vi "Pusher_Client_SetHandler.vi"(6 "_data":T1, 8 "ErrIn":errorcluster, 9 "Debug(F)":bool, 11 "Client in":refnum<class "Client.lvclass">) -> (0 "ErrOut":errorcluster, 2 "Path":path, 3 "Client out":refnum<class "Client.lvclass">)   [LabVIEW 2009, in "Client.lvclass"]
uses:
  Client.lvclass
  Pusher_Client_MonitorData.ctl
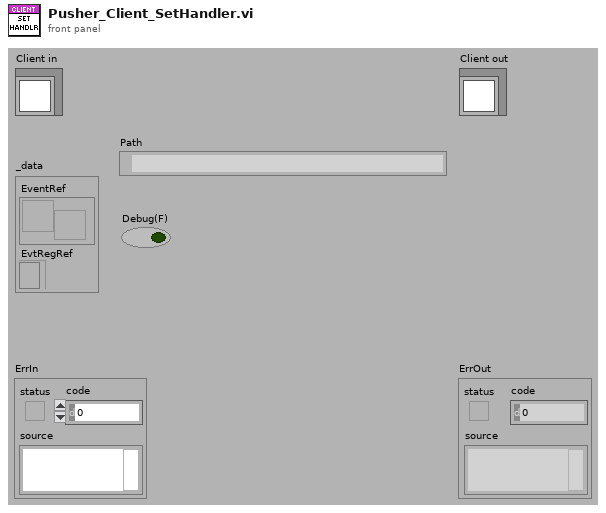
[diagram p1: front panel]
types:
  T1 = typedef "Client.lvclass/Pusher_Client_MonitorData.ctl" = cluster{"EventRef":refnum<user-event>, "EvtRegRef":refnum<event-registration>}
  T2 = enum32{"Invalid", "Standard", "Closed", "Hidden", "Minimized", "Maximized"}
  T3 = enum32{"Bad", "Idle", "Run top level", "Running"}[]
  T4 = enum32{"Bad", "Idle", "Run top level", "Running"}
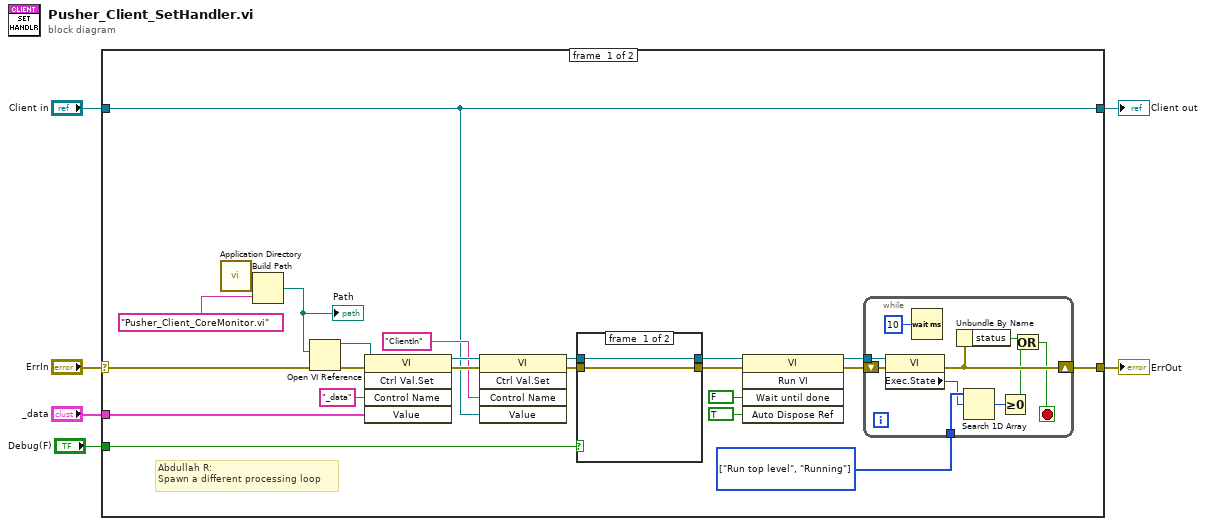
[diagram p0: block diagram]
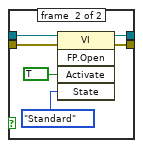
[diagram p2: hidden frame]
diagram:
  n1 = case shown="No Error" "ErrIn" {
    selector: "ErrIn" -> [w29 w49]
    tunnel: [w14 w49] -> w5
    tunnel: [w10 w48] -> w3
    tunnel: "Client in" -> [w10 w48]
    tunnel: "_data" -> [w20 _]
    tunnel: "Debug(F)" -> [w17 _]
    frame #0 {
      w9 = T3 [enum."Run top level", enum."Running"] items=["Bad", "Idle", "Run top level", "Running"]
      # "Abdullah R:\nSpawn a different processing loop"
      n2 = call <vilib>:"Application Directory.vi"() -> ("Application Directory"=w28:path)
      n3 = Build Path(base path=w28, name or relative path="Pusher_Client_CoreMonitor.vi") -> (appended path=w26:path)
      "Path" <- w26
      n4 = Open VI Reference(vi path=w26, error in (no error)=w29) -> (vi reference=w24:refnum<vi>, error out=w25:errorcluster)  [unwired: 4 in]
      n5 = invoke class="VI" method="Ctrl Val.Set"(reference=w24, error in=w25, "Control Name"="_data", "Value"=w20) -> (reference out=w12:refnum<vi>, error out=w13:errorcluster)  [unwired: 1 in, 3 out]
      n6 = invoke class="VI" method="Ctrl Val.Set"(reference=w12, error in=w13, "Control Name"="ClientIn", "Value"=w10) -> (reference out=w7:refnum<vi>, error out=w8:errorcluster)  [unwired: 1 in, 3 out]
      n7 = case shown="True" w17 {
        tunnel: w7 -> [w41 w47]
        tunnel: w8 -> [w40 w46]
        tunnel: [w40 w43] -> w19
        tunnel: [w41 w42] -> w18
        frame #0 {
        }
        frame #1 {
          n8 = invoke class="VI" method="FP.Open"(reference=w47, error in=w46, "Activate"=TRUE ("Activate?"), "State"=T2."Standard") -> (reference out=w42:refnum<vi>, error out=w43:errorcluster)  [unwired: 1 in, 3 out]
        }
      }
      n9 = invoke class="VI" method="Run VI"(reference=w18, error in=w19, "Wait until done"=FALSE ("Wait Until Done"), "Auto Dispose Ref"=TRUE ("Auto Dispose Reference")) -> (reference out=w15:refnum<vi>, error out=w16:errorcluster)  [unwired: 1 in, 3 out]
      n10 = while {
        tunnel: w15 -> [w38]
        tunnel: w9 -> [w33]
        shift-right: [w36] -> w14
        shift-left: w16 -> [w39]
        stop <- w34 stop-if-true
        n11 = property class="VI"(reference=w38, error in=w39) -> (error out=w36:errorcluster, "Exec.State"=w32:T4)  [unwired: 1 out]
        n12 = Wait (ms)(milliseconds to wait=u32 10) -> ()  [unwired: 1 out]
        n13 = Unbundle By Name(w36) -> ("status"=w35:bool)
        n14 = Search 1D Array(1D array=w33, element=w32) -> (index of element=w31:i32)  [unwired: 1 in]
        n15 = Greater Or Equal To 0?(x=w31) -> (x >= 0?=w30:bool)
        n16 = Or(x=w35, y=w30) -> (x .or. y?=w34:bool)
      }
    }
    frame #1 {
    }
  }
  "ErrOut" <- w5
  "Client out" <- w3
